vi "cblas zcopy.vi"(5 "n":i32=-1, 6 "incy":i32=1, 7 "incx":i32=1, 10 "y":cdb[](array[numeric]), 11 "x":cdb[](array[numeric])) -> (0 "error":i32, 3 "zcopy":cdb[](array[numeric]))   [LabVIEW 2020, in "NI_AALBLAS.lvlib"]
uses:
  NI_AALBLAS.lvlib
  <resource>/lvblas.dll
panel:
  # "void cblas_zcopy(n, *x, incx, *y, incy)"
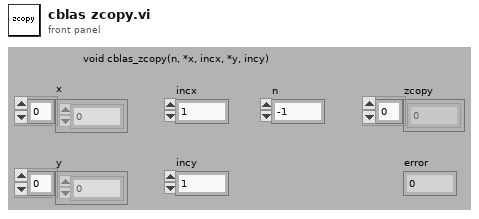
[diagram p1: front panel]
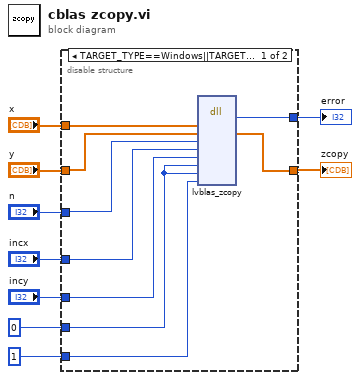
[diagram p0: block diagram]
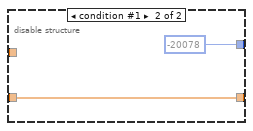
[diagram p2: hidden frame]
diagram:
  n1 = disable-structure shown="TARGET_TYPE==Windows||TARGET_TYPE==Unix||TARGET_TYPE==Mac||TARGET_TYPE==RT" {
    disable-tunnel: "y" -> [w17 w20]
    disable-tunnel: [w15 w20] -> w8
    disable-tunnel: [w16 -20078] -> w7
    disable-tunnel: "x" -> [w18 _]
    disable-tunnel: "n" -> [w14 _]
    disable-tunnel: 0 -> [w13 _]
    disable-tunnel: "incx" -> [w12 _]
    disable-tunnel: "incy" -> [w11 _]
    disable-tunnel: 1 -> [w10 _]
    frame condition #0 (active) {
      n2 = dll-call lib="C:/Program Files (x86)/National Instruments/LabVIEW 2020/resource/lvblas.*" fn="lvblas_zcopy" ("LVBLAS.dll:CxBLASCopyVectorH")("X"=w18, "Y"=w17, "N"=w14, "IncX"=w12, "IncY"=w11, "startX"=w13, "startY"=w13, "check"=w10) -> ("error"=w16:i32, "Y"=w15:cdb[])  [unwired: 10 in, 2 out]
    }
    frame condition #1 {
    }
  }
  "zcopy" <- w8
  "error" <- w7
